vi "Set Cell Type.vi"   [LabVIEW 2014]
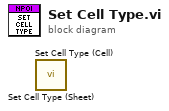
[diagram p0: block diagram]
diagram:
  n1 = call "Set Cell Type (Sheet).vi"() -> ()  [unwired: 10 in, 2 out]
  n2 = call "Set Cell Type (Cell).vi"() -> ()  [unwired: 10 in, 2 out]
